vi "PID_Implementation.vi"() -> ()   [LabVIEW 2022 SP3]
uses:
  <vilib>/MakerHub/LINX/Public/Sensors/Accelerometer/MPU60X0/DeviceAddresses.ctl
  <vilib>/MakerHub/LINX/Public/Sensors/Accelerometer/MPU60X0/AccelFullScaleRanges.ctl
  <vilib>/MakerHub/LINX/Public/Sensors/Accelerometer/MPU60X0/GyroFullScaleRanges.ctl
  <vilib>/MakerHub/LINX/Public/Peripherals/Digital/Digital Write N Chans.vi
  <vilib>/MakerHub/LINX/Private/Local IO/LinxDigitalWrite.vi
  <vilib>/MakerHub/LINX/Public/Utilities/Check Channel.vi
  <vilib>/MakerHub/LINX/Public/Utilities/Open Serial.vi
  <vilib>/MakerHub/LINX/Private/Utilties/Generate Error.vi
  <vilib>/MakerHub/LINX/Public/Peripherals/PWM/PWM Set Duty Cycle N Chans.vi
  <vilib>/MakerHub/LINX/LMH-LINX.lvlib
  <vilib>/MakerHub/LINX/Public/Sensors/Accelerometer/MPU60X0/MPU60X0.lvlib
panel:
  out "PID Values":dbl(graph)=0.030913936688571095
  out "Angle Reading":dbl(graph)=0.1713300456467663
  out "PID Value":dbl=0.030913936688571095
  in  "Kd":dbl=0.0005781
  in  "Ki":dbl=0.0286589
  in  "alpha":dbl=0.98
  in  "Baud Rate Override":u32=115200
  in  "Serial Port":refnum<visa-resource-name>="COM8"
  out "Acceleration Data (g)":T1={"X Axis"=480, "Y Axis"=2508, "Z Axis"=14508}
  in  "stop":bool
  out "angle rad":dbl=0.1713300456467663 format="%0.5f"
  in  "Offset":dbl=-377.638 format="%#_13g"
  out "Loop Rate (Hz)":u32=42
  in  "Kp":dbl=15.3286
  out "min(x,y)":dbl[](array[numeric])=[0.030913936688571095, 0.030913936688571095]
  in  "setpoint":dbl=0.182
  out "atan2(y,x)":dbl=0.17108655598022693
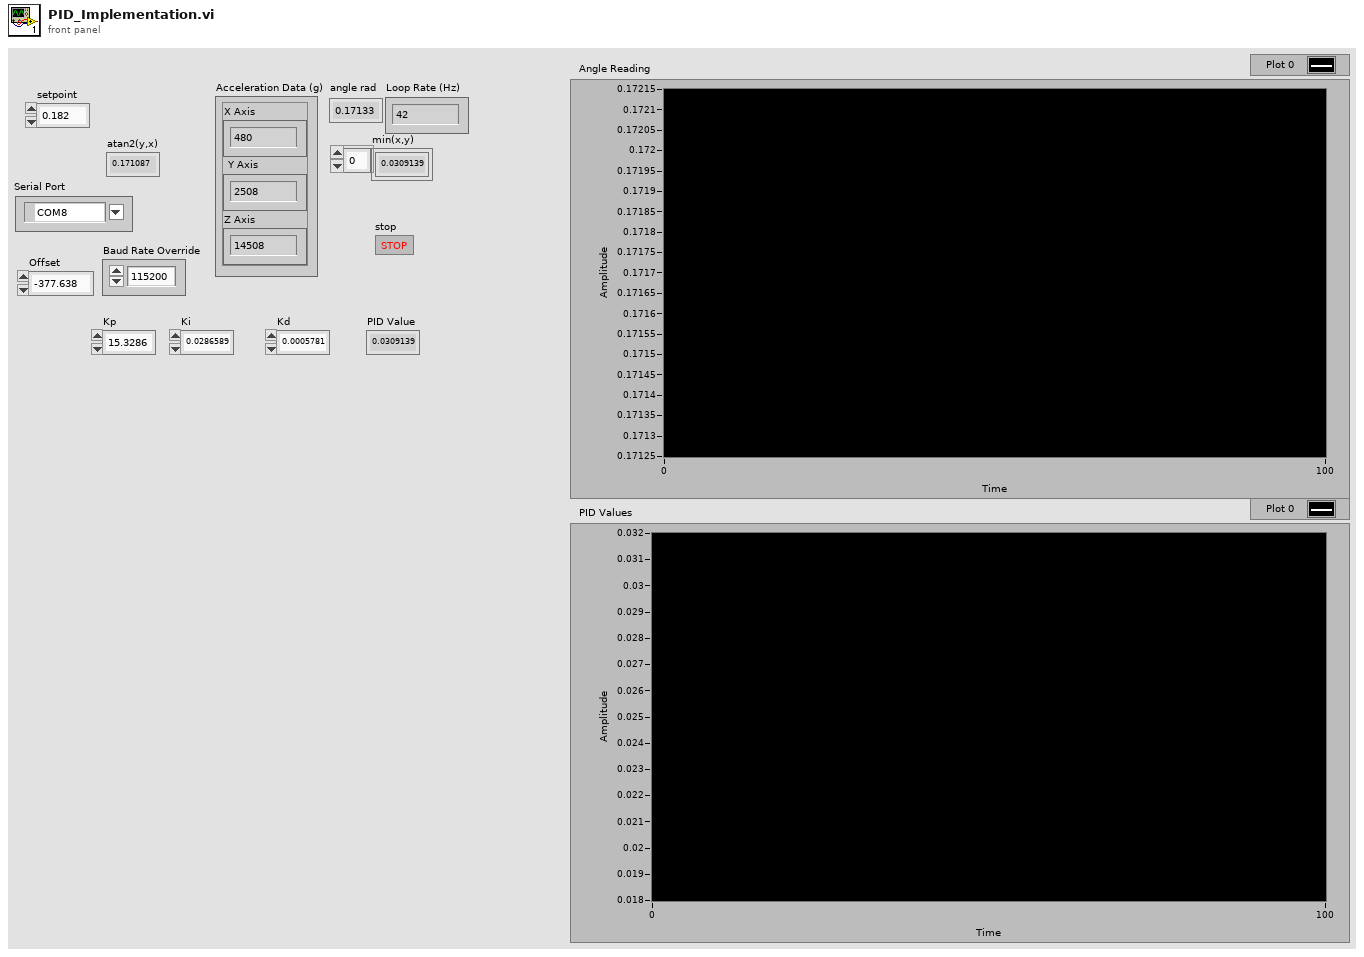
[diagram p1: front panel]
types:
  T1 = cluster{"X Axis":i16, "Y Axis":i16, "Z Axis":i16}
  T2 = typedef "LMH-LINX.lvlib/MPU60X0.lvlib/GyroFullScaleRanges.ctl" = enum8{"±250 °/s", "±500 °/s", "±1000 °/s", "±2000 °/s"}
  T3 = typedef "LMH-LINX.lvlib/MPU60X0.lvlib/AccelFullScaleRanges.ctl" = enum16{"±2g", "±4g", "±8g", "±16g"}
  T4 = typedef "LMH-LINX.lvlib/MPU60X0.lvlib/DeviceAddresses.ctl" = enum16{"0x68", "0x69"}
  T5 = typedef "LMH-LINX.lvlib/LINX Ref.ctl" = cluster{"IO":T6, "Interface":T7, "LINX Device Config":T8}
  T6 = typedef "LMH-LINX.lvlib/Platform.ctl" = enum16{"Remote", "Local"}
  T7 = typedef "LMH-LINX.lvlib/Interface.ctl" = enum16{"Serial", "TCP"}
  T8 = typedef "LMH-LINX.lvlib/Device.lvlib/LINX Device Config.ctl" = cluster{"Interface":T7, "COM Port":refnum<visa-resource-name>, "TCP Configuration":T9, "Device Family":u8, "Device ID":u8, "Device Name":string, "TCP Ref":refnum<k5>, "Channels":T10}
  T9 = typedef "LMH-LINX.lvlib/Device.lvlib/TCP Config.ctl" = cluster{"IP Address":string, "Port":u16}
  T10 = typedef "LMH-LINX.lvlib/Channels.ctl" = cluster{"DI":u8[], "DO":u8[], "AI":u8[], "AO":u8[], "PWM":u8[], "QE":u8[], "UART":u8[], "I2C 2":u8[], "SPI":u8[], "CAN":u8[], "Servo":u8[], "AI Ref (V)":dbl, "AI Resolution (Bits)":u8, "AO Ref (V)":dbl, "AO Resolution (Bits)":u8}
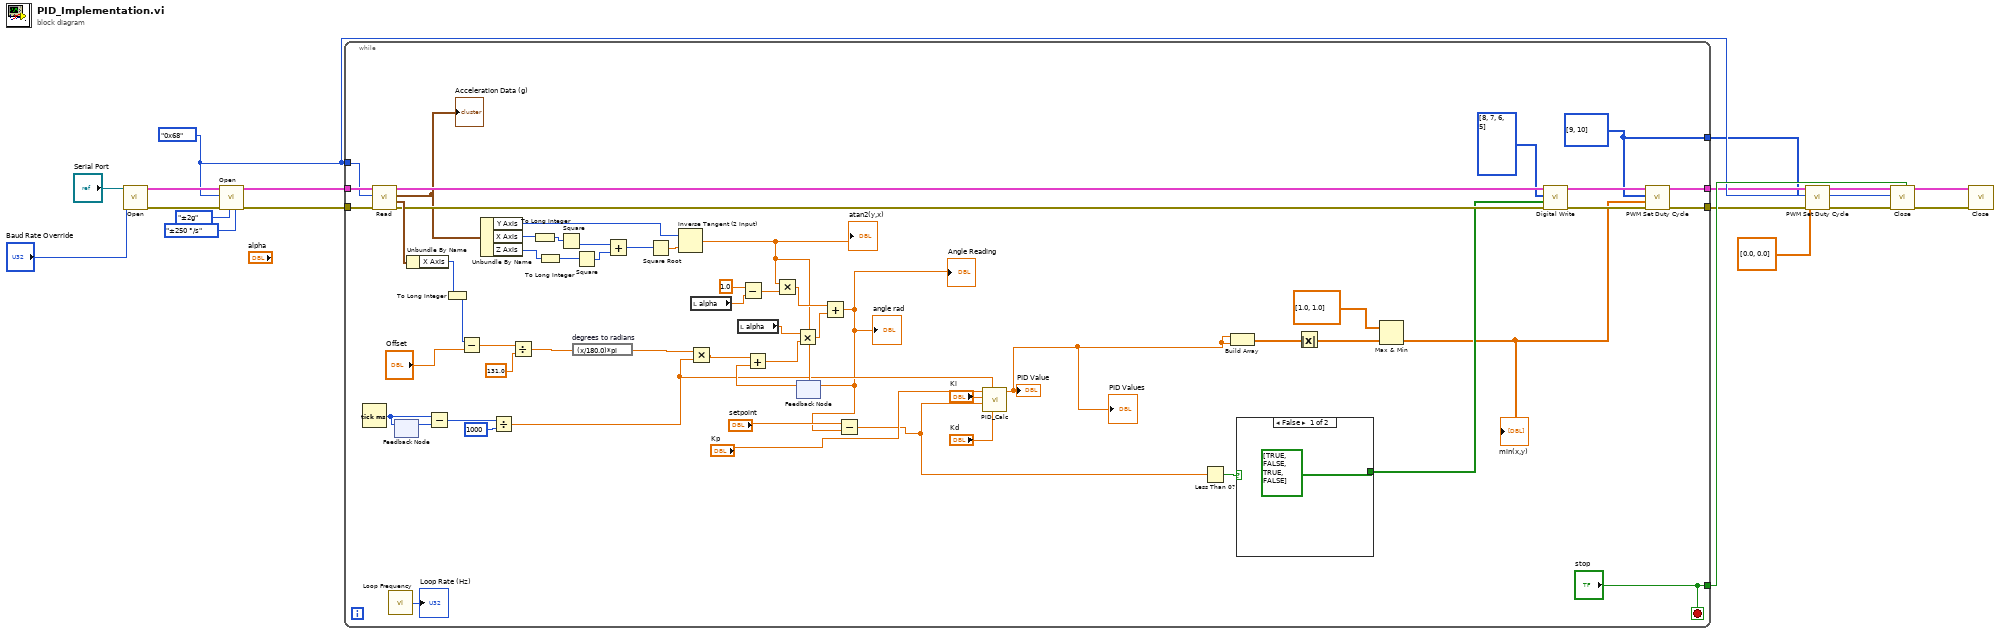
[diagram p0: block diagram]
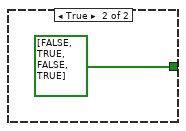
[diagram p2: hidden frame]
diagram:
  w7 = DeviceAddresses."0x68" ("I2C Slave Address")
  n1 = call-poly <vilib>:"Open.vi"("Baud Rate Override"="Baud Rate Override", "Serial Port"="Serial Port") -> ("Error Out"=w13:errorcluster, "LINX Resource"=w18:T5)  [unwired: 7 in, 1 out]
  n2 = call <vilib>:"Open.vi"("Gyro Full Scale Range"=GyroFullScaleRanges."±250 °/s", "Accel Full Scale Range"=AccelFullScaleRanges."±2g", "Error In"=w13, "I2C Slave Address"=w7, "LINX Resource"=w18) -> ("Error Out"=w14:errorcluster, "LINX Resource Out"=w17:T5)  [unwired: 5 in]
  n3 = while {
    tunnel: w17 -> [w77]
    tunnel: [w63] -> w6
    tunnel: [w62] -> w5
    tunnel: w14 -> [w76]
    tunnel: w7 -> [w75]
    tunnel: ["stop"] -> w8
    tunnel: [w27] -> w2
    stop <- "stop" stop-if-true
    w27 = u8[] [9, 10] ("PWM Channels")
    n4 = Tick Count (ms)() -> (millisecond timer value=w70:u32)
    n5 = call <vilib>:"Read.vi"("Error In"=w76, "I2C Slave Address"=w75, "LINX Resource"=w77) -> ("Error Out"=w60:errorcluster, "Gyro  Data (dps)"=w74:T1, "Acceleration Data (g)"=w50:T1, "LINX Resource Out"=w65:T5)  [unwired: 4 in, 1 out]
    "Acceleration Data (g)" <- w50
    n6 = call <vilib>:"Loop Frequency.vi"() -> ("Loop Rate (Hz)"=→"Loop Rate (Hz)":u32)
    n7 = feedback-in #1(w70) -> ()
    n8 = feedback #1() -> (w69:u32)  [unwired: 1 in]
    n9 = Unbundle By Name(w74) -> ("X Axis"=w58:i16)
    n10 = Subtract(x=w70, y=w69) -> (x-y=w68:u32)
    n11 = To Long Integer(number=w58) -> (32bit integer=w26:i32)
    n12 = Subtract(x=w26, y="Offset") -> (x-y=w72:dbl)
    n13 = Unbundle By Name(w50) -> ("Y Axis"=w41:i16, "X Axis"=w40:i16, "Z Axis"=w39:i16)
    n14 = Divide(x=w68, y=u32 1000) -> (x/y=w23:dbl)
    n15 = Divide(x=w72, y=131.0) -> (x/y=w51:dbl)
    n16 = To Long Integer(number=w40) -> (32bit integer=w34:i32)
    n17 = To Long Integer(number=w39) -> (32bit integer=w33:i32)
    n18 = Square(x=w34) -> (x^2=w38:i32)
    n19 = expression code="(x/180.0)*pi" "degrees to radians"(w51) -> (w32:dbl)
    n20 = Square(x=w33) -> (x^2=w37:i32)
    n21 = Add(x=w38, y=w37) -> (x+y=w36:i32)
    n22 = Square Root(x=w36) -> (sqrt(x)=w35:dbl)
    n23 = Inverse Tangent (2 Input)(1:w35, 2:w41) -> (0:w31:dbl)
    "atan2(y,x)" <- w31
    n24 = Multiply(x=w32, y=w23) -> (x*y=w30:dbl)
    n25 = local read "alpha"() -> (w48:dbl)
    n26 = local read "alpha"() -> (w46:dbl)
    n27 = Subtract(x=1.0, y=w48) -> (x-y=w47:dbl)
    n28 = Multiply(x=w31, y=w47) -> (x*y=w45:dbl)
    n29 = feedback #2(w31) -> (w29:dbl)
    n30 = Add(x=w30, y=w29) -> (x+y=w28:dbl)
    n31 = Multiply(x=w46, y=w28) -> (x*y=w44:dbl)
    n32 = Add(x=w45, y=w44) -> (x+y=w20:dbl)
    "angle rad" <- w20
    "Angle Reading" <- w20
    n33 = feedback-in #2(w20) -> ()
    n34 = Subtract(x="setpoint", y=w20) -> (x-y=w24:dbl)
    n35 = call "PID_Calc.vi"("Kd"="Kd", "dt"=w23, "Error Signal"=w24, "Ki"="Ki", "Kp"="Kp") -> ("PID Value"=w19:dbl)  [unwired: 6 in]
    "PID Value" <- w19
    "PID Values" <- w19
    n36 = Less Than 0?(x=w24) -> (x < 0?=w57:bool)
    n37 = Build Array(w19, w19) -> (w55:dbl[])
    n38 = case shown="False" w57 {
      tunnel: [bool[] [TRUE, FALSE, TRUE, FALSE] ("Values") bool[] [FALSE, TRUE, FALSE, TRUE] ("Values")] -> w56
      frame False {
      }
      frame True {
      }
    }
    n39 = Absolute Value(x=w55) -> (abs(x)=w54:dbl[])
    n40 = Max & Min(x=dbl[] [1.0, 1.0], y=w54) -> (min(x,y)=w52:dbl[])  [unwired: 1 out]
    "min(x,y)" <- w52
    n41 = call-poly <vilib>:"Digital Write.vi"("Error In"=w60, "Values"=w56, "DO Channels"=u8[] [8, 7, 6, 5], "LINX Resource"=w65) -> ("Error Out"=w61:errorcluster, "LINX Resource Out"=w64:T5)  [unwired: 6 in]
    n42 = call-poly <vilib>:"PWM Set Duty Cycle.vi"("Error In"=w61, "Duty Cycles"=w52, "PWM Channels"=w27, "LINX Resource"=w64) -> ("Error Out"=w62:errorcluster, "LINX Resource Out"=w63:T5)  [unwired: 6 in]
  }
  n43 = call-poly <vilib>:"PWM Set Duty Cycle.vi"("Error In"=w5, "Duty Cycles"=dbl[] [0.0, 0.0], "PWM Channels"=w2, "LINX Resource"=w6) -> ("Error Out"=w3:errorcluster, "LINX Resource Out"=w4:T5)  [unwired: 6 in]
  n44 = call <vilib>:"Close.vi"("Close I2C Master?"=w8, "Error In"=w3, "I2C Slave Address (0)"=w7, "LINX Resource"=w4) -> ("Error Out"=w15:errorcluster, "LINX Resource out"=w16:T5)  [unwired: 6 in]
  n45 = call <vilib>:"Close.vi"("Error In"=w15, "LINX Resource"=w16) -> ()  [unwired: 9 in, 1 out]
